vi "Test_RouteGuide_RequestStreaming.vi"() -> (0 "Array of Error Description":T1)   [LabVIEW 2019]
uses:
  gRPC_ATS/TestUtility/utility.llb/array of error description.ctl
  gRPC_ATS/TestUtility/utility.llb/error description.ctl
  gRPC_ATS/TestUtility/utility.llb/error type.ctl
  examples/route_guide/route_guide_client/RPC Messages/routeguide_RouteSummary.ctl
  examples/route_guide/route_guide_client/route_guide_client.lvlib
panel:
  out "Pass":bool
  in  "Client VI Path":path=path "../../examples/route_guide/route_guide_client/RequestStreaming RouteGuide Test.vi"
  in  "Server VI path":path=path "../../examples/route_guide/route_guide_server/Run Service.vi"
  in  "error in":errorcluster
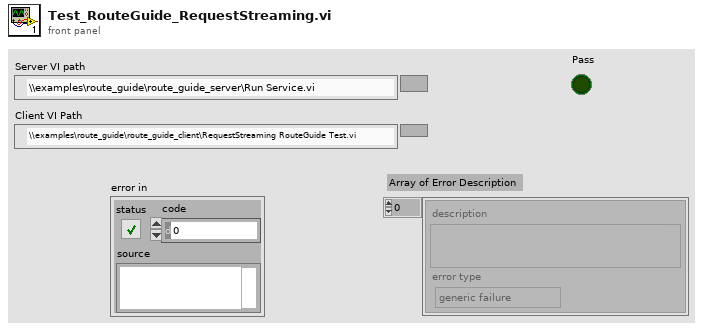
[diagram p1: front panel]
types:
  T1 = typedef "array of error description.ctl" = T2[]
  T2 = typedef "error description.ctl" = cluster{"description":string, "error type":T3}
  T3 = typedef "error type.ctl" = enum32{"generic failure", "boundary case", "precision", "expected error"}
  T4 = typedef "route_guide_client.lvlib/routeguide_RouteSummary.ctl" = cluster{"point_count":i32, "feature_count":i32, "distance":i32, "elapsed_time":i32}
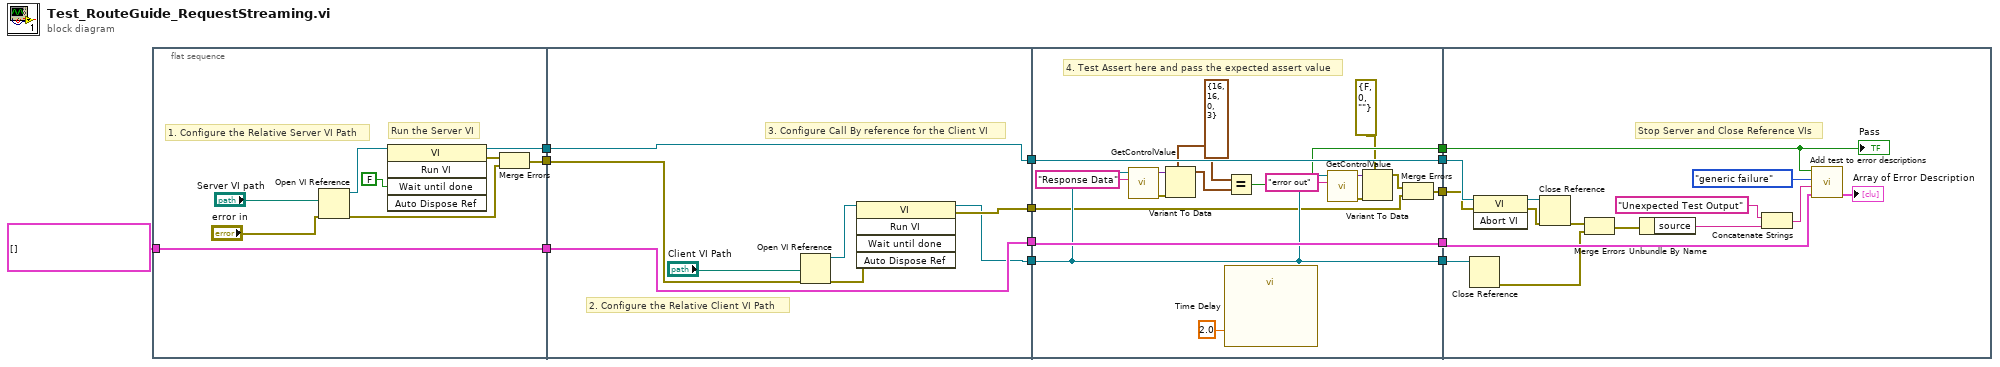
[diagram p0: block diagram]
diagram:
  n1 = flat-sequence {
    tunnel: T1 [] ("error descriptions in") -> [w18]
    tunnel: [w18] -> w13
    tunnel: [w17] -> w12
    tunnel: [w14] -> w11
    tunnel: w13 -> [w29]
    tunnel: [w29] -> w10
    tunnel: [w24] -> w9
    tunnel: [w28] -> w8
    tunnel: w12 -> [w28]
    tunnel: w11 -> [w27]
    tunnel: [w23] -> w2
    tunnel: w10 -> [w47]
    tunnel: [w47] -> w7
    tunnel: w9 -> [w32]
    tunnel: [w31] -> w6
    tunnel: [w46] -> w5
    tunnel: w8 -> [w46]
    tunnel: [w45] -> w3
    tunnel: w2 -> [w38]
    tunnel: [w38] -> w1
    tunnel: w7 -> [w57]
    tunnel: w6 -> [w53]
    tunnel: w5 -> [w54]
    tunnel: w3 -> [w52]
    tunnel: w1 -> [w51]
    frame #0 {
      # "1. Configure the Relative Server VI Path"
      # "Run the Server VI"
      n2 = Open VI Reference(vi path="Server VI path", error in (no error)="error in") -> (vi reference=w20:refnum<vi>, error out=w16:errorcluster)  [unwired: 4 in]
      n3 = invoke class="VI" method="Run VI"(reference=w20, "Wait until done"=FALSE ("Wait Until Done")) -> (reference out=w17:refnum<vi>, error out=w15:errorcluster)  [unwired: 3 in, 3 out]
      n4 = Merge Errors(w15, w16) -> (w14:errorcluster)
    }
    frame #1 {
      # "2. Configure the Relative Client VI Path"
      # "3. Configure Call By reference for the Client VI"
      n5 = Open VI Reference(vi path="Client VI Path", error in (no error)=w27) -> (vi reference=w25:refnum<vi>, error out=w26:errorcluster)  [unwired: 4 in]
      n6 = invoke class="VI" method="Run VI"(reference=w25, error in=w26) -> (reference out=w23:refnum<vi>, error out=w24:errorcluster)  [unwired: 3 in, 3 out]
    }
    frame #2 {
      w40 = T4 {"point_count"=16, "feature_count"=16, "distance"=0, "elapsed_time"=3} ("Response Data")
      # "4. Test Assert here and pass the expected assert value"
      n7 = call "GetControlValue.vi"("Control Label"="Response Data", "VI Reference"=w38) -> ("error out"=w42:errorcluster, "Value"=w41:variant)  [unwired: 8 in]
      n8 = Variant To Data(error in=w42, type=w40, Variant=w41) -> (data=w39:T4)  [unwired: 1 out]
      n9 = call "Time Delay"("Delay Time (s)"=2.0) -> ()  [unwired: 10 in, 1 out]
      n10 = Equal?(x=w40, y=w39) -> (x = y?=w45:bool)
      n11 = call "GetControlValue.vi"("Control Label"="error out", "VI Reference"=w38) -> ("error out"=w36:errorcluster, "Value"=w35:variant)  [unwired: 8 in]
      n12 = Variant To Data(error in=w36, type=errorcluster {"status"=FALSE, "code"=0, "source"=""} ("error constant"), Variant=w35) -> (data=w33:errorcluster)  [unwired: 1 out]
      n13 = Merge Errors(w33, w32) -> (w31:errorcluster)
    }
    frame #3 {
      # "Stop Server and Close Reference VIs"
      n14 = Close Reference(reference=w51) -> (error out=w49:errorcluster)  [unwired: 1 in]
      n15 = invoke class="VI" method="Abort VI"(reference=w54, error in=w53) -> (reference out=w55:refnum<vi>, error out=w56:errorcluster)  [unwired: 1 in, 1 out]
      n16 = Close Reference(reference=w55, error in (no error)=w56) -> (error out=w50:errorcluster)
      n17 = Merge Errors(w50, w49) -> (w48:errorcluster)
      n18 = Unbundle By Name(w48) -> ("source"=w59:string)
      n19 = Concatenate Strings("Unexpected Test Output" ("string"), w59) -> (w60:string)
      n20 = call "Add test to error descriptions.vi"("error descriptions in"=w57, "error string"=w60, "error type"=error_type."generic failure", "pass"=w52) -> ("error description out"=→"Array of Error Description":T1)  [unwired: 3 in]
      "Pass" <- w52
    }
  }
